vi "UpdateUI.vi"(1 "LabramHR References":T2, 2 "Acquisition Settings":T1) -> ()   [LabVIEW 2014]
uses:
  Spectrometer Refnum.ctl
  Measurements/Plot Data/Optical Spectrum Plot Refnum.ctl
  Laser.ctl
  Filter.ctl
  Grating.ctl
  Detector.ctl
  Acquisition Settings.ctl
panel:
  # "LICENSED MATERIALS – PROPERTY OF IBM\nCopyright IBM Corp. 2016,\nALL RIGHTS RESERVED"
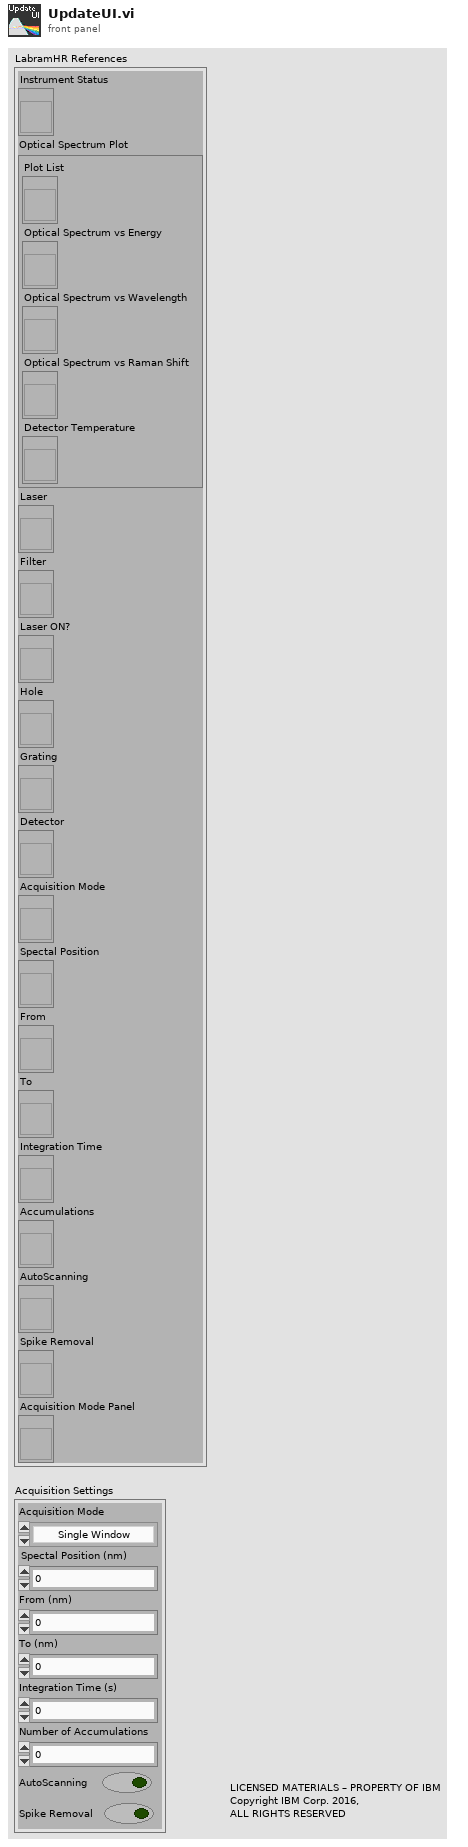
[diagram p1: front panel]
types:
  T1 = typedef "Acquisition Settings.ctl" = cluster{"Acquisition Mode":enum16{"Single Window", "Multi-Window"}, "Spectal Position (nm)":dbl, "From (nm)":dbl, "To (nm)":dbl, "Integration Time (s)":dbl, "Number of Accumulations":i32, "AutoScanning":bool, "Spike Removal":bool}
  T2 = typedef "Spectrometer Refnum.ctl" = cluster{"Instrument Status":refnum<vi>, "Optical Spectrum Plot":T3, "Laser":refnum<vi>, "Filter":refnum<vi>, "Laser ON?":refnum<vi>, "Hole":refnum<vi>, "Grating":refnum<vi>, "Detector":refnum<vi>, "Acquisition Mode":refnum<vi>, "Spectal Position":refnum<vi>, "From":refnum<vi>, "To":refnum<vi>, "Integration Time":refnum<vi>, "Accumulations":refnum<vi>, "AutoScanning":refnum<vi>, "Spike Removal":refnum<vi>, "Acquisition Mode Panel":refnum<vi>}
  T3 = typedef "Optical Spectrum Plot Refnum.ctl" = cluster{"Plot List":refnum<vi>, "Optical Spectrum vs Energy":refnum<vi>, "Optical Spectrum vs Wavelength":refnum<vi>, "Optical Spectrum vs Raman Shift":refnum<vi>, "Detector Temperature":refnum<vi>}
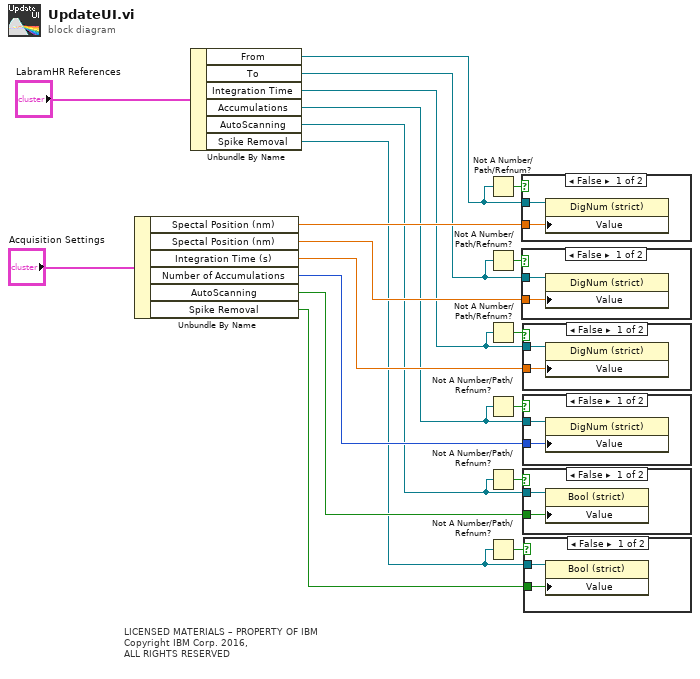
[diagram p0: block diagram]
diagram:
  # "LICENSED MATERIALS – PROPERTY OF IBM\nCopyright IBM Corp. 2016,\nALL RIGHTS RESERVED"
  n1 = Unbundle By Name("Acquisition Settings") -> ("Spectal Position (nm)"=w20:dbl, "Spectal Position (nm)"=w17:dbl, "Integration Time (s)"=w16:dbl, "Number of Accumulations"=w15:i32, "AutoScanning"=w14:bool, "Spike Removal"=w13:bool)
  n2 = Unbundle By Name("LabramHR References") -> ("From"=w6:refnum<vi>, "To"=w5:refnum<vi>, "Integration Time"=w4:refnum<vi>, "Accumulations"=w3:refnum<vi>, "AutoScanning"=w2:refnum<vi>, "Spike Removal"=w1:refnum<vi>)
  n3 = Not A Number/Path/Refnum?(number/path/refnum=w6) -> (NaN/Path/Refnum?=w12:bool)
  n4 = Not A Number/Path/Refnum?(number/path/refnum=w5) -> (NaN/Path/Refnum?=w11:bool)
  n5 = Not A Number/Path/Refnum?(number/path/refnum=w4) -> (NaN/Path/Refnum?=w10:bool)
  n6 = Not A Number/Path/Refnum?(number/path/refnum=w3) -> (NaN/Path/Refnum?=w9:bool)
  n7 = Not A Number/Path/Refnum?(number/path/refnum=w2) -> (NaN/Path/Refnum?=w8:bool)
  n8 = Not A Number/Path/Refnum?(number/path/refnum=w1) -> (NaN/Path/Refnum?=w7:bool)
  n9 = case shown="False" w12 {
    tunnel: w20 -> [w22 _]
    tunnel: w6 -> [w21 _]
    frame False {
      n10 = property class="DigNum (strict)"(reference=w21, "Value"=w22) -> ()  [unwired: 1 in, 2 out]
    }
    frame True {
    }
  }
  n11 = case shown="False" w11 {
    tunnel: w5 -> [w24 _]
    tunnel: w17 -> [w23 _]
    frame False {
      n12 = property class="DigNum (strict)"(reference=w24, "Value"=w23) -> ()  [unwired: 1 in, 2 out]
    }
    frame True {
    }
  }
  n13 = case shown="False" w10 {
    tunnel: w4 -> [w26 _]
    tunnel: w16 -> [w25 _]
    frame False {
      n14 = property class="DigNum (strict)"(reference=w26, "Value"=w25) -> ()  [unwired: 1 in, 2 out]
    }
    frame True {
    }
  }
  n15 = case shown="False" w9 {
    tunnel: w3 -> [w28 _]
    tunnel: w15 -> [w27 _]
    frame False {
      n16 = property class="DigNum (strict)"(reference=w28, "Value"=w27) -> ()  [unwired: 1 in, 2 out]
    }
    frame True {
    }
  }
  n17 = case shown="False" w8 {
    tunnel: w2 -> [w30 _]
    tunnel: w14 -> [w29 _]
    frame False {
      n18 = property class="Bool (strict)"(reference=w30, "Value"=w29) -> ()  [unwired: 1 in, 2 out]
    }
    frame True {
    }
  }
  n19 = case shown="False" w7 {
    tunnel: w1 -> [w32 _]
    tunnel: w13 -> [w31 _]
    frame False {
      n20 = property class="Bool (strict)"(reference=w32, "Value"=w31) -> ()  [unwired: 1 in, 2 out]
    }
    frame True {
    }
  }
